vi "Read Service.vi"(8 "error in (no error)":errorcluster, 11 "Manejo Turnos in":refnum<class "Manejo Turnos.lvclass">) -> (0 "error out":errorcluster, 3 "Manejo Turnos out":refnum<class "Manejo Turnos.lvclass">)   [LabVIEW 2020, in "Manejo Turnos.lvlib" / "Manejo Turnos.lvclass"]
uses:
  Manejo Turnos.lvclass
  Manejo Turnos.lvclass/Manejo Turnos.ctl
  <vilib>/drjdpowell/SQLite Library/SQL Connection/Open (path).vi
  <vilib>/drjdpowell/SQLite Library/SQL Connection/Open (string).vi
  <vilib>/AdvancedString/Path To Command Line String.vi
  <vilib>/drjdpowell/SQLite Library/SQL Connection/Execute SQL.vi
  <vilib>/drjdpowell/SQLite Library/SQL Connection/Connection.lvclass
  <vilib>/drjdpowell/SQLite Library/SQLite.lvlib
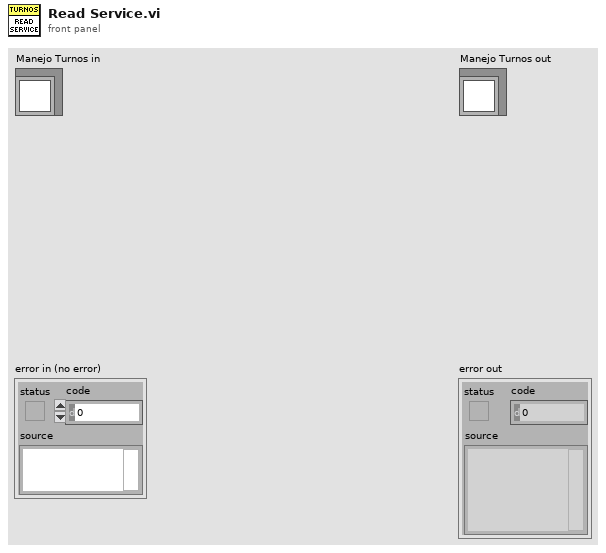
[diagram p1: front panel]
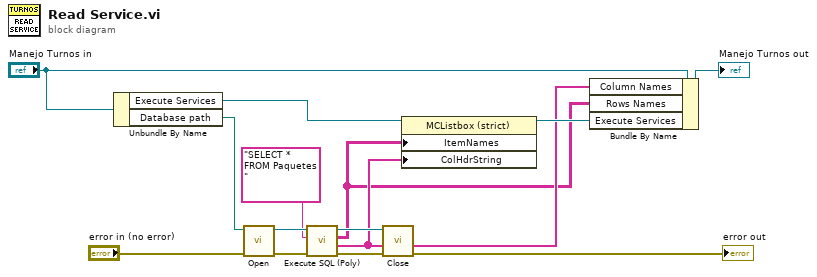
[diagram p0: block diagram]
diagram:
  n1 = Unbundle By Name("Manejo Turnos in") -> ("Execute Services"=w4:refnum<vi>, "Database path"=w10:path)
  n2 = call-poly <vilib>:"Open.vi"("error in (no error)"="error in (no error)", "db file"=w10) -> ("error out"=w13:errorcluster, "SQLite Connection"=w9:refnum<class "Connection.lvclass">)  [unwired: 8 in]
  n3 = call-poly <vilib>:"Execute SQL (Poly).vi"("error in (no error)"=w13, "SQL"="SELECT * FROM Paquetes ", "SQLite Connection in"=w9) -> ("error out"=w14:errorcluster, "Column Names"=w2:string[], "Result Set"=w1:string[][], "SQLite Connection"=w8:refnum<class "Connection.lvclass">)  [unwired: 5 in]
  n4 = call-dynamic "Close.vi"("error in (no error)"=w14, "SQLite Connection in"=w8) -> ("error out"=→"error out":errorcluster)  [unwired: 9 in]
  n5 = property class="MCListbox (strict)"(reference=w4, "ItemNames"=w1, "ColHdrString"=w2) -> (reference out=w3:refnum<vi>)  [unwired: 1 in, 1 out]
  n6 = Bundle By Name(cluster="Manejo Turnos in", "Column Names"=w2, "Rows Names"=w1, "Execute Services"=w3) -> (→"Manejo Turnos out":refnum<class "Manejo Turnos.lvclass">)
